vi "Config dialog.vi"(8 "error in (no error)":errorcluster, 11 "DAQ config params in":T1={"DAQ Device Name"="Dev2", "Physical channel"=""}) -> (0 "error out":errorcluster, 2 "Cancelled?":bool, 3 "DAQ config params out":T1={"DAQ Device Name"="Dev2", "Physical channel"=""})   [LabVIEW 2020]
uses:
  controls/Config dialog states -- enum.ctl
  <resource>/objmgr/daqmx.rc
  controls/DAQ config parameters -- cluster.ctl
panel:
  out "DAQ config params (old)":T1={"DAQ Device Name"="Dev2", "Physical channel"=""}
  in  "Analog input":u16(ring) items=["Dev1/ai0", "Dev1/ai1", "Dev1/ai2", "Dev1/ai3", "Dev1/ai4", "Dev1/ai5", "Dev1/ai6", "Dev1/ai7", "Dev1/ai8", "Dev1/ai9", "Dev1/ai10", "Dev1/ai11", "Dev1/ai12", "Dev1/ai13", "Dev1/ai14", "Dev1/ai15"]
  in  "Cancel":bool
  in  "OK":bool
  in  "DAQ Device Name":tag
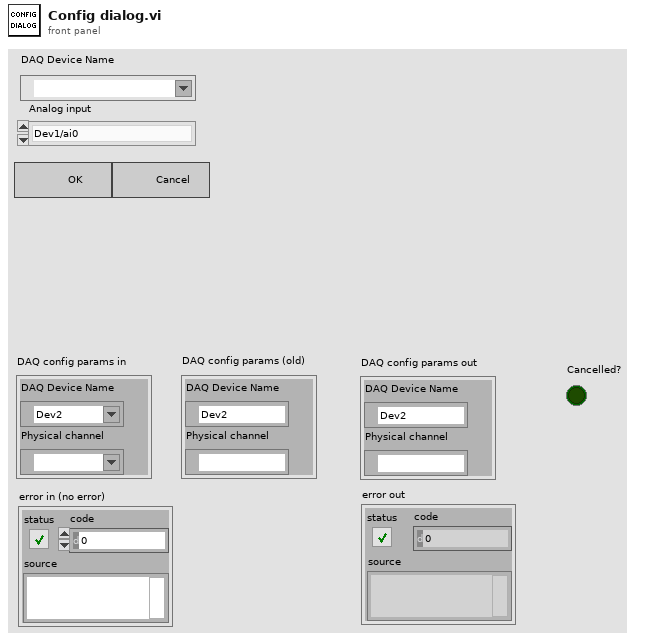
[diagram p1: front panel]
types:
  T1 = typedef "DAQ config parameters -- cluster.ctl" = cluster{"DAQ Device Name":tag, "Physical channel":tag}
  T2 = typedef "Config dialog states -- enum.ctl" = enum16{"Wait", "Initialize", "Update data", "Exit"}
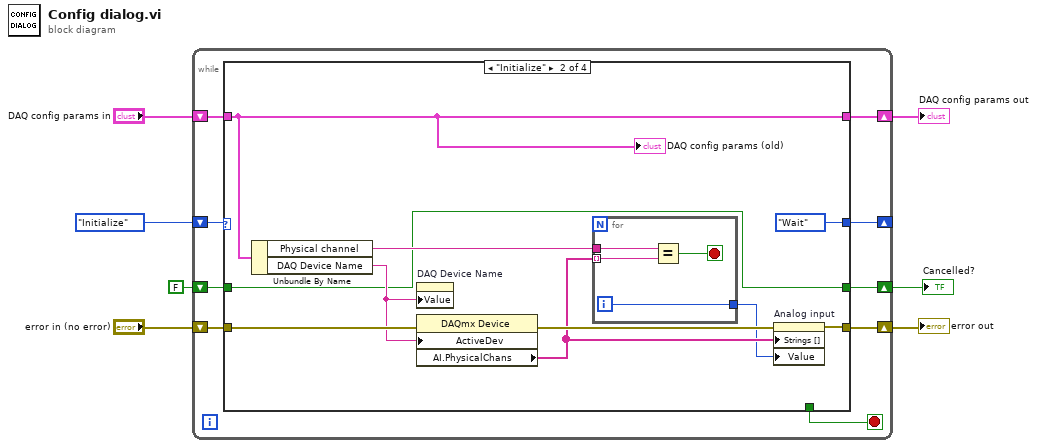
[diagram p0: block diagram]
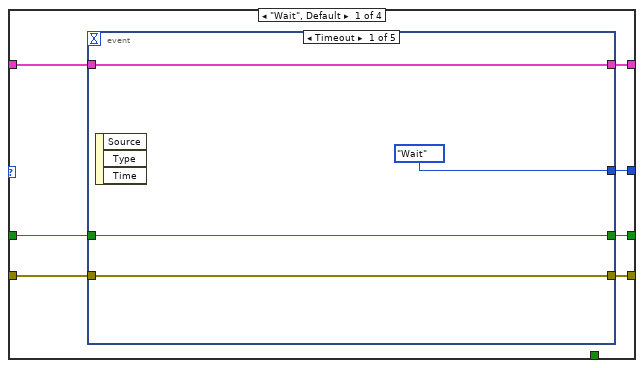
[diagram p2: hidden frame]
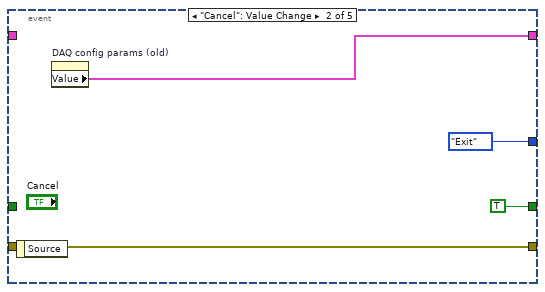
[diagram p3: hidden frame]
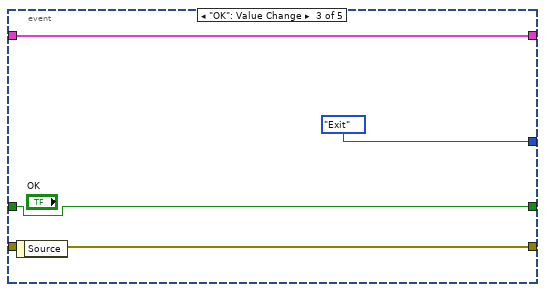
[diagram p4: hidden frame]
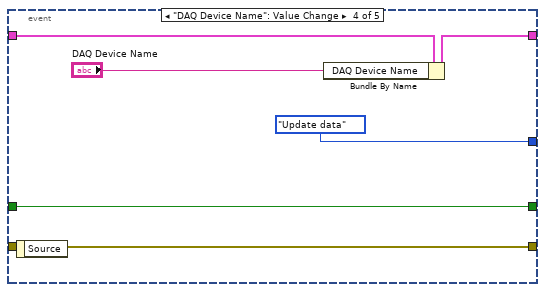
[diagram p5: hidden frame]
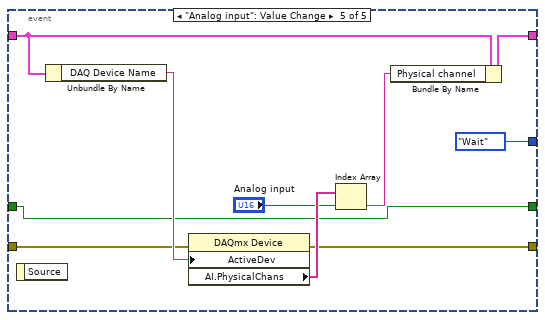
[diagram p6: hidden frame]
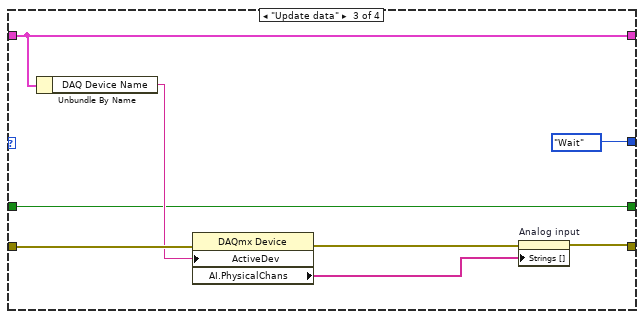
[diagram p7: hidden frame]
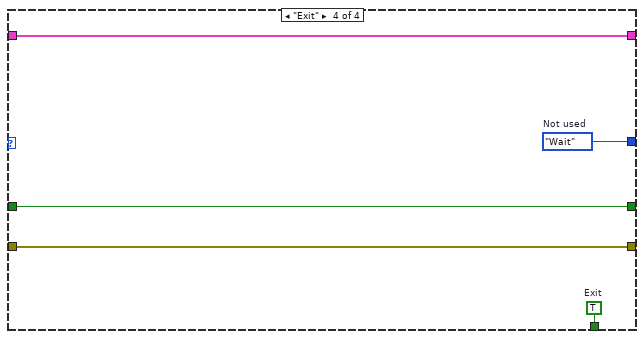
[diagram p8: hidden frame]
diagram:
  n1 = while {
    shift-right: [w14] -> _
    shift-left: Config_dialog_states_--_enum."Initialize" -> [w16]
    shift-right: [w12] -> w5
    shift-left: "error in (no error)" -> [w13]
    shift-right: [w10] -> w3
    shift-left: "DAQ config params in" -> [w11]
    shift-right: [w9] -> w2
    shift-left: FALSE -> [w8]
    stop <- w15 stop-if-true
    n2 = case shown="\"Initialize\"" w16 {
      tunnel: [_ _ _ w78] -> w15
      tunnel: [w23 Config_dialog_states_--_enum."Wait" ("Not used") Config_dialog_states_--_enum."Wait" ("Not used") w77] -> w14
      tunnel: w13 -> [w20 w60 w70 w76]
      tunnel: [w19 w58 w69 w76] -> w12
      tunnel: w11 -> [w22 w57 w68 w75]
      tunnel: [w21 w57 w68 w75] -> w10
      tunnel: [w18 w52 w66 w74] -> w9
      tunnel: w8 -> [w17 w52 w66 w74]
      frame "Wait", Default {
        n3 = event shown="[0] Timeout" {
          selector: _ -> [_ _ _ _ _]
          dyn-events: _ -> [_ _ _ _ _]
          timeout: _ -> [_ _ _ _ _]
          tunnel: [Config_dialog_states_--_enum."Wait" Config_dialog_states_--_enum."Exit" Config_dialog_states_--_enum."Exit" Config_dialog_states_--_enum."Update data" Config_dialog_states_--_enum."Wait"] -> w23
          tunnel: w22 -> [w26 _ w34 w41 w50]
          tunnel: [w26 w30 w34 w39 w51] -> w21
          tunnel: w20 -> [w25 w29 w33 w37 w48]
          tunnel: [w25 w29 w33 w37 w43] -> w19
          tunnel: [w24 TRUE w32 w36 w42] -> w18
          tunnel: w17 -> [w24 _ w32 w36 w42]
          event Timeout {
            n4 = event-data() -> ()  [unwired: 1 in, 3 out]
          }
          event "Cancel": Value Change {
            n5 = event-data() -> ()  [unwired: 1 in, 1 out]
            n6 = property on="DAQ config params (old)" class="Clust (strict)"() -> ("Value"=w30:T1)  [unwired: 2 in, 2 out]
          }
          event "OK": Value Change {
            n7 = event-data() -> ()  [unwired: 1 in, 1 out]
          }
          event "DAQ Device Name": Value Change {
            n8 = event-data() -> ()  [unwired: 1 in, 1 out]
            n9 = Bundle By Name(cluster=w41, "DAQ Device Name"="DAQ Device Name") -> (w39:T1)
          }
          event "Analog input": Value Change {
            n10 = event-data() -> ()  [unwired: 1 in, 1 out]
            n11 = Unbundle By Name(w50) -> ("DAQ Device Name"=w49:tag)
            n12 = property class="DAQmx Device"(error in=w48, "ActiveDev"=w49) -> (error out=w43:errorcluster, "AI.PhysicalChans"=w47:tag[])  [unwired: 1 in, 1 out]
            n13 = Index Array(array=w47, index="Analog input") -> (element=w45:tag)
            n14 = Bundle By Name(cluster=w50, "Physical channel"=w45) -> (w51:T1)
          }
        }
      }
      frame "Initialize" {
        n15 = Unbundle By Name(w57) -> ("Physical channel"=w53:tag, "DAQ Device Name"=w56:tag)
        n16 = property on="DAQ Device Name" class="DAQmxName"("Value"=w56) -> ()  [unwired: 2 in, 2 out]
        n17 = property class="DAQmx Device"(error in=w60, "ActiveDev"=w56) -> (error out=w59:errorcluster, "AI.PhysicalChans"=w55:tag[])  [unwired: 1 in, 1 out]
        n18 = for {
          tunnel: w55 -> [w63] mode=indexing
          tunnel: w53 -> [w64]
          tunnel: [w65] -> w54
          i -> [w65]
          stop <- w62 stop-if-true
          n19 = Equal?(x=w64, y=w63) -> (x = y?=w62:bool)
        }
        n20 = property on="Analog input" class="Ring (strict)"(error in=w59, "Strings []"=w55, "Value"=w54) -> (error out=w58:errorcluster)  [unwired: 1 in, 1 out]
        "DAQ config params (old)" <- w57
      }
      frame "Update data" {
        n21 = Unbundle By Name(w68) -> ("DAQ Device Name"=w67:tag)
        n22 = property class="DAQmx Device"(error in=w70, "ActiveDev"=w67) -> (error out=w72:errorcluster, "AI.PhysicalChans"=w71:tag[])  [unwired: 1 in, 1 out]
        n23 = property on="Analog input" class="Ring (strict)"(error in=w72, "Strings []"=w71) -> (error out=w69:errorcluster)  [unwired: 1 in, 1 out]
      }
      frame "Exit" {
        w77 = Config_dialog_states_--_enum."Wait"  # Not used
        w78 = TRUE  # Exit
      }
    }
  }
  "error out" <- w5
  "DAQ config params out" <- w3
  "Cancelled?" <- w2
